vi "SecurityAccess_sendKey.vi"(8 "error in (no error)":errorcluster, 9 "SecuritySeed":u16 format="%.0x", 10 "subFunction":T1=2 items=["SPSsendKey"=2, "DevCtrlsendKey"=4], 11 "diag ref in":T2) -> (0 "error out":errorcluster, 1 "success?":bool, 3 "diag ref out":T2)   [LabVIEW 2013, in "GMLAN.lvlib"]
uses:
  GMLAN.lvlib
  <vilib>/Automotive Diagnostic Command Set/Diagnostic Transport.llb/Diag Reference.ctl
  <vilib>/Automotive Diagnostic Command Set/Diagnostic Transport.llb/Transport Protocol Selector.ctl
  <vilib>/Automotive Diagnostic Command Set/Diagnostic Transport.llb/Diag CAN Frame Log.ctl
  SecurityAccess_sendKey_SubFunctions.ctl
  <vilib>/addons/Automotive Diagnostic Command Set/NI_Automotive Diagnostic Command Set.lvlib
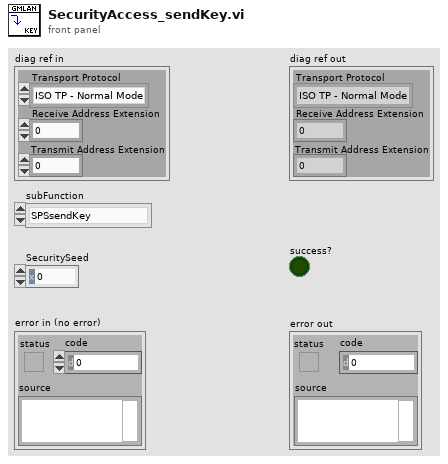
[diagram p1: front panel]
types:
  T1 = typedef "GMLAN.lvlib/SecurityAccess_sendKey_SubFunctions.ctl" = u8
  T2 = typedef "NI_Automotive Diagnostic Command Set.lvlib/Diag Reference.ctl" = cluster{"Diag CAN Handle":u32, "Transport Protocol":T3, "Receive Address Extension":u8, "Transmit Address Extension":u8, "Receive CAN Id":u32, "Transmit CAN Id":u32, "Diag CAN Queue":refnum<queue>, "Log Frames ?":bool, "My TP Address":u8, "Other TP Address":u8, "T1":u16, "T2":u16, "T3":u16, "T4":u16, "Tx SN":u8, "Block Size":u8, "Rx SN":u8, "VW TP Initialized?":bool, "Tx block no":u8, "baud rate":u32, "Interface":string, "Channel Diag CAN Handle":u32, "UDP Connection ID":refnum<k16>, "TCP Connection ID":refnum<k5>, "Target IP Addr":u32, "Source Address":u16, "Target Address":u16, "Send Header NACK?":bool, "DLL Handle":u32, "NAD":u8}
  T3 = typedef "NI_Automotive Diagnostic Command Set.lvlib/Transport Protocol Selector.ctl" = enum16{"ISO TP - Normal Mode", "ISO TP - Mixed Mode", "VW TP 2.0", "Diagnostics on IP", "ISO TP LIN"}
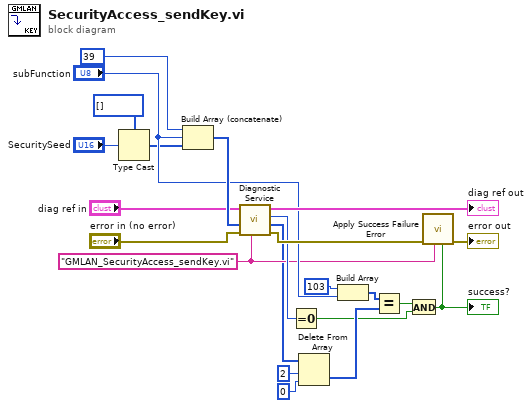
[diagram p0: block diagram]
diagram:
  w5 = "GMLAN_SecurityAccess_sendKey.vi" ("error source")
  n1 = Type Cast(type=u8[] [], x="SecuritySeed") -> (*(type *) &x=w1:u8[])
  n2 = Build Array (concatenate)(u8 39 ("element"), "subFunction", w1) -> (w18:T1[])
  n3 = call <vilib>:"Diagnostic Service.vi"("error source"=w5, "error in (no error)"="error in (no error)", "data in"=w18, "diag ref in"="diag ref in") -> ("error out"=w20:errorcluster, "data out"=w4:u8[], "error code"=w16:u8, "diag ref out"=→"diag ref out":T2)  [unwired: 2 in, 2 out]
  n4 = Equal To 0?(x=w16) -> (x = 0?=w10:bool)
  n5 = Delete From Array(array=w4, length=2, index=0) -> (deleted portion=w11:u8[])  [unwired: 1 out]
  n6 = Build Array(u8 103 ("element"), "subFunction") -> (w12:T1[])
  n7 = Equal?(x=w12, y=w11) -> (x = y?=w9:bool)
  n8 = And(x=w9, y=w10) -> (x .and. y?=w6:bool)
  "success?" <- w6
  n9 = call <vilib>:"Apply Success Failure Error.vi"("success code"=w6, "error source"=w5, "error in (no error)"=w20) -> ("error out"=→"error out":errorcluster)  [unwired: 8 out]
